vi "Get Terminal Subaddress.vi"(8 "error in":errorcluster, 11 "subaddress in":T2 format="%.0x") -> (0 "error out":errorcluster, 2 "subaddress value":T1, 3 "subaddress out":T2 format="%.0x", 4 "found?":bool)   [LabVIEW 2020, in "AIM MIL-STD-1553 Scripting.lvlib"]
uses:
  AIM MIL-STD-1553 Scripting.lvlib
  <vilib>/NI VeriStand/Custom Device API/Custom Device Item Ref.ctl
  Shared/Address.ctl
  Constants.vi
  <vilib>/NI VeriStand/Custom Device API/Get Item Property (U16).vi
  <vilib>/NI VeriStand/Custom Device API/Custom Device API.lvlib
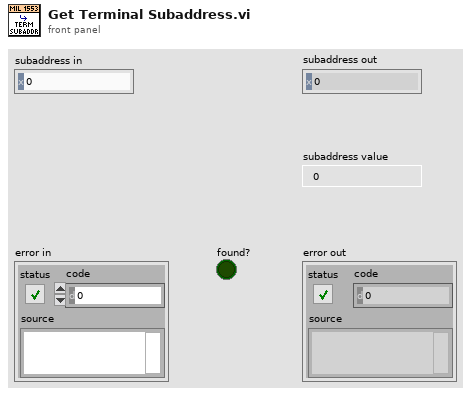
[diagram p1: front panel]
types:
  T1 = typedef "Address.ctl" = u16
  T2 = typedef "Custom Device API.lvlib/Custom Device Item Ref.ctl" = u64
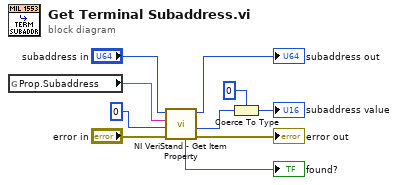
[diagram p0: block diagram]
diagram:
  n1 = global read "Constants.vi" "Prop.Subaddress"() -> (w6:string)
  n2 = call-poly <vilib>:"NI VeriStand - Get Item Property.vi"("error in (no error)"="error in", "Default Value"=u16 0 ("subaddress"), "Property Name"=w6, "Item Ref in"="subaddress in") -> ("error out"=→"error out":errorcluster, "Value"=w2:u16, "Item Ref out"=→"subaddress out":T2, "Found?"=→"found?":bool)  [unwired: 4 in]
  n3 = Coerce To Type(0:w2, 1:T1 0 ("terminal address")) -> (2:→"subaddress value":T1)
